vi "Find Variable Value If Operands are Equal.vi"(0 "Monkey":string, 1 "Monkeys":T1, 2 "Variable":string) -> (3 "Variable Value":u64)   [LabVIEW 2020, in "AoC 2022.lvlib"]
uses:
  AoC 2022.lvlib
  Day 11 - Monkey in the Middle/private/Monkeys.ctl
  Day 11 - Monkey in the Middle/private/Monkey.ctl
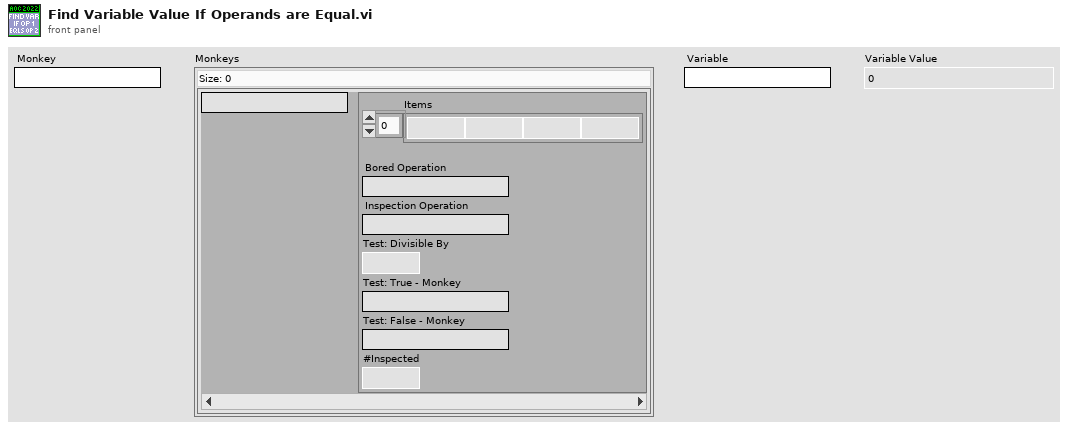
[diagram p1: front panel]
types:
  T1 = typedef "AoC 2022.lvlib/Monkeys.ctl" = map{string, T2}
  T2 = typedef "AoC 2022.lvlib/Monkey.ctl" = cluster{"Items":u64[], "Bored Operation":string, "Inspection Operation":string, "Test: Divisible By":u64, "Test: True - Monkey":string, "Test: False - Monkey":string, "#Inspected":i32}
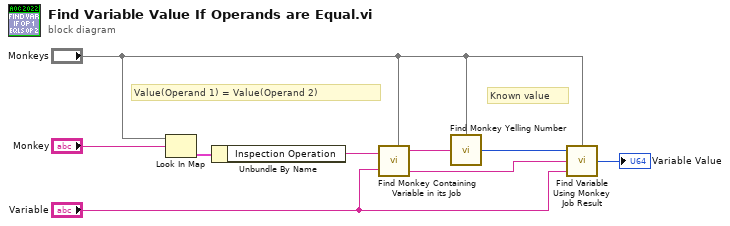
[diagram p0: block diagram]
diagram:
  # "Known value"
  # "Value(Operand 1) = Value(Operand 2)"
  n1 = Look In Map(map="Monkeys", key="Monkey") -> (value=w8:T2)  [unwired: 1 in, 1 out]
  n2 = Unbundle By Name(w8) -> ("Inspection Operation"=w9:string)
  n3 = call "Find Monkey Containing Variable in its Job.vi"("Monkeys"="Monkeys", "Variable"="Variable", "Monkey Job Statement"=w9) -> ("Monkey having Variable in its Job"=w5:string, "Monkey not having Variable in its Job"=w6:string)  [unwired: 2 out]
  n4 = call "Find Monkey Yelling Number.vi"("Monkey"=w6, "Monkeys"="Monkeys") -> ("Monkey Yelling Number"=w3:u64)
  n5 = call "Find Variable Using Monkey Job Result.vi"("Monkeys"="Monkeys", "Variable"="Variable", "Monkey"=w5, "Job Result"=w3) -> ("Variable Value"=→"Variable Value":u64)
